vi "cRIO Daten estmalig an PC uebergeben.vi"(8 "Fehler (Eingang)":errorcluster) -> (0 "Fehler (Ausgang)":errorcluster)   [LabVIEW 2020, in "Kommunikation mit cRIO.lvlib"]
uses:
  Kommunikation mit cRIO.lvlib
  Seiten/Anlagengrenzwerte/FGV Anlagengrenzwerte Aktionen.ctl
  Seiten/Erweiterte Konfig/FGV PID Aktionen.ctl
  Seiten/Anlagengrenzwerte/Anlagengrenzwerte.lvlib
  Seiten/Erweiterte Konfig/Erweiterte Konfig.lvlib
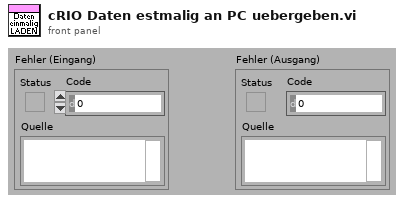
[diagram p1: front panel]
types:
  T1 = typedef "Erweiterte Konfig.lvlib/FGV PID Aktionen.ctl" = enum16{"Lesen", "Schreiben PID", "Schreiben Sonstige", "Dichtheitstest", "Aktionen Dicht.", "Parameter Sensor"}
  T2 = typedef "Anlagengrenzwerte.lvlib/FGV Anlagengrenzwerte Aktionen.ctl" = enum16{"Lesen", "Grenzwerte schreiben"}
  T3 = cluster{"Array[0]":sgl, "Array[1]":sgl, "Array[2]":sgl, "Array[3]":sgl, "Array[4]":sgl}
  T4 = cluster{"Array[0]":sgl, "Array[1]":sgl, "Array[2]":sgl, "Array[3]":sgl, "Array[4]":sgl, "Array[5]":sgl}
  T5 = cluster{"Array[0]":sgl, "Array[1]":sgl, "Array[2]":sgl, "Array[3]":sgl, "Array[4]":sgl, "Array[5]":sgl, "Array[6]":sgl, "Array[7]":sgl, "Array[8]":sgl, "Array[9]":sgl}
  T6 = cluster{"[0]":cluster{"Array[0]":sgl, "Array[1]":sgl, "Array[2]":sgl, "Array[3]":sgl, "Array[4]":sgl}, "[1]":cluster{"Array[0]":sgl, "Array[1]":sgl, "Array[2]":sgl, "Array[3]":sgl, "Array[4]":sgl}, "[2]":cluster{"Array[0]":sgl, "Array[1]":sgl, "Array[2]":sgl, "Array[3]":sgl, "Array[4]":sgl}, "[3]":cluster{"Array[0]":sgl, "Array[1]":sgl, "Array[2]":sgl, "Array[3]":sgl, "Array[4]":sgl}, "[4]":cluster{"Array[0]":sgl, "Array[1]":sgl, "Array[2]":sgl, "Array[3]":sgl, "Array[4]":sgl}}
  T7 = cluster{"Array[0]":sgl, "Array[1]":sgl, "Array[2]":sgl, "Array[3]":sgl, "Array[4]":sgl, "Array[5]":sgl, "Array[6]":sgl, "Array[7]":sgl, "Array[8]":sgl, "Array[9]":sgl, "Array[10]":sgl, "Array[11]":sgl, "Array[12]":sgl, "Array[13]":sgl, "Array[14]":sgl, "Array[15]":sgl, "Array[16]":sgl, "Array[17]":sgl, "Array[18]":sgl, "Array[19]":sgl}
  T8 = cluster{"[0]":cluster{"Array[0]":sgl, "Array[1]":sgl, "Array[2]":sgl, "Array[3]":sgl, "Array[4]":sgl, "Array[5]":sgl}, "[1]":cluster{"Array[0]":sgl, "Array[1]":sgl, "Array[2]":sgl, "Array[3]":sgl, "Array[4]":sgl, "Array[5]":sgl}, "[2]":cluster{"Array[0]":sgl, "Array[1]":sgl, "Array[2]":sgl, "Array[3]":sgl, "Array[4]":sgl, "Array[5]":sgl}, "[3]":cluster{"Array[0]":sgl, "Array[1]":sgl, "Array[2]":sgl, "Array[3]":sgl, "Array[4]":sgl, "Array[5]":sgl}, "[4]":cluster{"Array[0]":sgl, "Array[1]":sgl, "Array[2]":sgl, "Array[3]":sgl, "Array[4]":sgl, "Array[5]":sgl}, "[5]":cluster{"Array[0]":sgl, "Array[1]":sgl, "Array[2]":sgl, "Array[3]":sgl, "Array[4]":sgl, "Array[5]":sgl}, "[6]":cluster{"Array[0]":sgl, "Array[1]":sgl, "Array[2]":sgl, "Array[3]":sgl, "Array[4]":sgl, "Array[5]":sgl}, "[7]":cluster{"Array[0]":sgl, "Array[1]":sgl, "Array[2]":sgl, "Array[3]":sgl, "Array[4]":sgl, "Array[5]":sgl}, "[8]":cluster{"Array[0]":sgl, "Array[1]":sgl, "Array[2]":sgl, "Array[3]":sgl, "Array[4]":sgl, "Array[5]":sgl}, "[9]":cluster{"Array[0]":sgl, "Array[1]":sgl, "Array[2]":sgl, "Array[3]":sgl, "Array[4]":sgl, "Array[5]":sgl}, "[10]":cluster{"Array[0]":sgl, "Array[1]":sgl, "Array[2]":sgl, "Array[3]":sgl, "Array[4]":sgl, "Array[5]":sgl}, "[11]":cluster{"Array[0]":sgl, "Array[1]":sgl, "Array[2]":sgl, "Array[3]":sgl, "Array[4]":sgl, "Array[5]":sgl}, "[12]":cluster{"Array[0]":sgl, "Array[1]":sgl, "Array[2]":sgl, "Array[3]":sgl, "Array[4]":sgl, "Array[5]":sgl}, "[13]":cluster{"Array[0]":sgl, "Array[1]":sgl, "Array[2]":sgl, "Array[3]":sgl, "Array[4]":sgl, "Array[5]":sgl}}
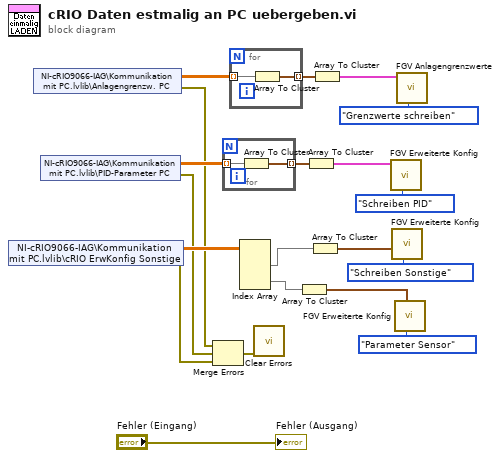
[diagram p0: block diagram]
diagram:
  n1 = shared-variable "NI-cRIO9066-IAG\\Kommunikation mit PC.lvlib\\cRIO ErwKonfig Sonstige"() -> (w10:sgl[][], error out=w6:errorcluster)  [unwired: 1 in]
  n2 = shared-variable "NI-cRIO9066-IAG\\Kommunikation mit PC.lvlib\\Anlagengrenzw. PC"() -> (w14:sgl[][], error out=w8:errorcluster)  [unwired: 1 in]
  n3 = shared-variable "NI-cRIO9066-IAG\\Kommunikation mit PC.lvlib\\PID-Parameter PC"() -> (w12:sgl[][], error out=w7:errorcluster)  [unwired: 1 out]
  n4 = Merge Errors(w8, w7, w6) -> (w5:errorcluster)
  n5 = for {
    tunnel: w12 -> [w21] mode=indexing
    tunnel: [w22] -> w16 mode=indexing
    n6 = Array To Cluster(array=w21) -> (cluster=w22:T3)
  }
  n7 = for {
    tunnel: w14 -> [w24] mode=indexing
    tunnel: [w23] -> w15 mode=indexing
    n8 = Array To Cluster(array=w24) -> (cluster=w23:T4)
  }
  n9 = Index Array(array=w10) -> (element #1=w4:sgl[], element #2=w3:sgl[])  [unwired: 4 in]
  n10 = call <vilib>:"Clear Errors.vi"("error in (no error)"=w5) -> ()  [unwired: 5 in, 2 out]
  n11 = Array To Cluster(array=w3) -> (cluster=w1:T5)
  n12 = Array To Cluster(array=w16) -> (cluster=w11:T6)
  n13 = Array To Cluster(array=w4) -> (cluster=w9:T7)
  n14 = Array To Cluster(array=w15) -> (cluster=w13:T8)
  n15 = call "FGV Erweiterte Konfig.vi"("Aktion"=FGV_PID_Aktionen."Schreiben PID", "PID-Parameter Anzeige"=w11) -> ()  [unwired: 4 in, 6 out]
  n16 = call "FGV Erweiterte Konfig.vi"("Aktion"=FGV_PID_Aktionen."Schreiben Sonstige", "Sonstige"=w9) -> ()  [unwired: 4 in, 6 out]
  n17 = call "FGV Erweiterte Konfig.vi"("Aktion"=FGV_PID_Aktionen."Parameter Sensor", "Parameter Sensoren"=w1) -> ()  [unwired: 4 in, 6 out]
  n18 = call "FGV Anlagengrenzwerte.vi"("Aktion"=FGV_Anlagengrenzwerte_Aktionen."Grenzwerte schreiben", "Anlagen-Grenzwerte Anzeige"=w13) -> ()  [unwired: 9 in, 1 out]
  "Fehler (Ausgang)" <- "Fehler (Eingang)"
